vi "macro_TrajectoryConstraint_RectRegion.vi"   [LabVIEW 2019, in "Trajectory_Library.lvlib"]
uses:
  Trajectory_Library.lvlib
types:
  T1 = typedef "Trajectory_Library.lvlib/TRANSLATION2D.ctl" = cluster{"X":dbl, "Y":dbl}
  T2 = typedef "Trajectory_Library.lvlib/TRAJ_CONSTRAINT_MAX_VELOCITY.ctl" = cluster{"Max Velocity":dbl, "IM UNIQUE":bool}
  T3 = typedef "Trajectory_Library.lvlib/TRAJ_CONSTRAINT_RECT_REGION.ctl" = cluster{"BottomLeftPoint":T1, "TopRightPoint":T1, "Constraint":variant, "Constraint Type":T4}
  T4 = typedef "Trajectory_Library.lvlib/TRAJ_CONSTRAINT_TYPES_ENUM.ctl" = enum16{"UNDEFINED", "DIFF DRIVE KINEMATICS", "DIFF DRIVE VOLTAGE", "CENTRIPITAL ACCEL", "MECA DRIVE KINEMATICS", "SWERVE DRIVE KINEMATICS", "MAXIMUM VELOCITY", "ELLIPTICAL REGION", "RECTANGULAR REGION"}
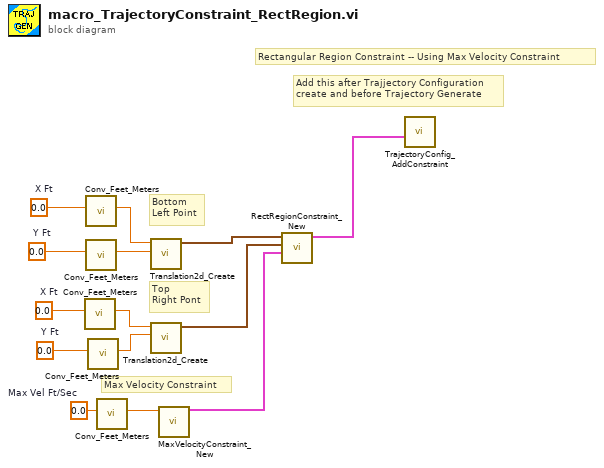
[diagram p0: block diagram]
diagram:
  w4 = 0.0  # Max Vel Ft/Sec
  w7 = 0.0  # X Ft
  w6 = 0.0  # Y Ft
  w11 = 0.0  # X Ft
  w10 = 0.0  # Y Ft
  # "Max Velocity Constraint"
  # "Bottom\nLeft Point"
  # "Top \nRight Pont"
  # "Rectangular Region Constraint -- Using Max Velocity Constraint"
  # "Add this after Trajjectory Configuration\ncreate and before Trajectory Generate"
  n1 = call "Conv_Feet_Meters.vi"("Feet"=w7) -> ("Meters"=w9:dbl)  [unwired: 10 in]
  n2 = call "Conv_Feet_Meters.vi"("Feet"=w11) -> ("Meters"=w13:dbl)  [unwired: 10 in]
  n3 = call "Conv_Feet_Meters.vi"("Feet"=w10) -> ("Meters"=w12:dbl)  [unwired: 10 in]
  n4 = call "Conv_Feet_Meters.vi"("Feet"=w6) -> ("Meters"=w8:dbl)  [unwired: 10 in]
  n5 = call "Conv_Feet_Meters.vi"("Feet"=w4) -> ("Meters"=w5:dbl)  [unwired: 10 in]
  n6 = call "Translation2d_Create.vi"("Y"=w12, "X"=w13) -> ("TRANSLATION"=w3:T1)  [unwired: 9 in]
  n7 = call "Translation2d_Create.vi"("Y"=w8, "X"=w9) -> ("TRANSLATION"=w2:T1)  [unwired: 9 in]
  n8 = call "MaxVelocityConstraint_New.vi"("Maximum Velocity"=w5) -> ("MAX_VELOCITY_CONSTRAINT"=w1:T2)  [unwired: 10 in]
  n9 = call "RectRegionConstraint_New.vi"("Constraint Data Cluster"=w1, "TopRightPoint"=w2, "BottomLeftPoint"=w3) -> ("RECT_REGION_CONSTRAINT"=w14:T3)  [unwired: 8 in]
  n10 = call "TrajectoryConfig_AddConstraint.vi"("Constraint"=w14) -> ()  [unwired: 10 in, 1 out]
